vi "Read.vi"(8 "error in":errorcluster, 11 "CANopen Master in":refnum<class "CANopen Master.lvclass">) -> (0 "error out":errorcluster, 1 "Empty?":bool, 2 "CANopen Message out":refnum<class "CANopen Response Message.lvclass">, 3 "CANopen Master out":refnum<class "CANopen Master.lvclass">)   [LabVIEW 2024, in "CANopen Master.lvlib" / "CANopen Master.lvclass"]
uses:
  CANopen Master.lvclass
  CANopen Response/CANopen Response Message.lvclass
  D:/git/CANopen-XNET/CANopen Message/CANopen Message.lvclass
  CANopen Master.lvclass/CANopen Master.ctl
  HAL/Source/Interfaces/ICommunicate/ICommunicate.lvclass
  HAL/Source/Interfaces/IMessage/IMessage.lvclass
  CANopen Message/CANopen Message.lvclass
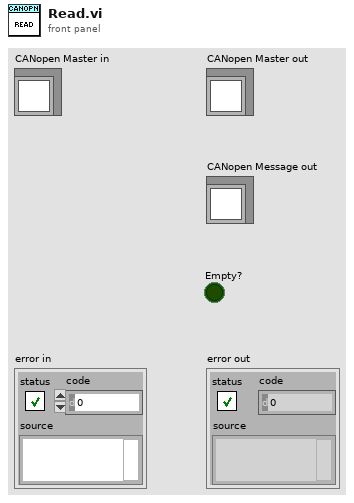
[diagram p1: front panel]
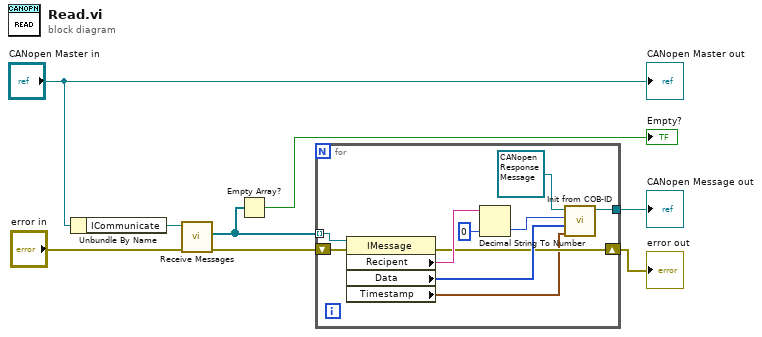
[diagram p0: block diagram]
diagram:
  n1 = Unbundle By Name("CANopen Master in") -> ("ICommunicate"=w6:refnum<class "ICommunicate.lvclass">)
  n2 = call-dynamic "Receive Messages.vi"("error in"="error in", "ICommunicate in"=w6) -> ("error out"=w4:errorcluster, "Messages"=w2:refnum<class "IMessage.lvclass">[])  [unwired: 7 in, 1 out]
  n3 = Empty Array?(array=w2) -> (empty?=→"Empty?":bool)
  n4 = for {
    tunnel: [w18] -> w7
    tunnel: w2 -> [w16] mode=indexing
    shift-right: [w10] -> w1
    shift-left: w4 -> [w15]
    n5 = property class="IMessage"(reference=w16, error in=w15) -> (error out=w10:errorcluster, "Recipent"=w13:string, "Data"=w14:u8[], "Timestamp"=w9:timestamp)  [unwired: 1 out]
    n6 = Decimal String To Number(string=w13, default (0L)=u32 0) -> (number=w12:u32)  [unwired: 1 in, 1 out]
    n7 = call "Init from COB-ID.vi"("Timestamp"=w9, "Data"=w14, "COB-ID"=w12, "CANopen Message in"=refnum<class "CANopen Response Message.lvclass"> refnum ("CANopen Master.lvlib:CANopen Request.lvclass")) -> ("CANopen Message out"=w18:refnum<class "CANopen Response Message.lvclass">)  [unwired: 7 in]
  }
  "error out" <- w1
  "CANopen Message out" <- w7
  "CANopen Master out" <- "CANopen Master in"
